vi "UHR-Fleezers Control (host) - 11.0.vi"() -> ()   [LabVIEW 2011] (continued)
                                }
                                frame #1 {
                                n486 = local read "Yank to which?"() -> (w782:bool)
                                n487 = case shown="False" w782 {
                                tunnel: w783 -> [_ w811]
                                tunnel: w781 -> [w784 _]
                                frame False {
                                n488 = flat-sequence {
                                tunnel: w784 -> [w785]
                                frame #0 {
                                n489 = property on="Trap Pos FB SP" class="DigNum (strict)"("Val(Sgnl)"=w785) -> ()  [unwired: 2 in, 2 out]
                                }
                                frame #1 {
                                n490 = Wait (ms)(milliseconds to wait=u32 700) -> ()  [unwired: 1 out]
                                }
                                frame #2 {
                                n491 = local read "Action (%)"() -> (w790:dbl)
                                n492 = Absolute Value(x=w790) -> (abs(x)=w789:dbl)
                                n493 = Greater?(x=w789, y=70.0) -> (0:w787:bool)
                                n494 = property on="Remove Action Offset" class="Bool (strict)"("Val(Sgnl)"=w787) -> ()  [unwired: 2 in, 2 out]
                                }
                                frame #3 {
                                n495 = for {
                                N: 4 -> [_]
                                n496 = flat-sequence {
                                frame #0 {
                                n497 = Wait (ms)(milliseconds to wait=u32 500) -> ()  [unwired: 1 out]
                                }
                                frame #1 {
                                n498 = local read "Action (%)"() -> (w796:dbl)
                                n499 = Absolute Value(x=w796) -> (abs(x)=w795:dbl)
                                n500 = Greater?(x=w795, y=70.0) -> (0:w793:bool)
                                n501 = property on="Remove Action Offset" class="Bool (strict)"("Val(Sgnl)"=w793) -> ()  [unwired: 2 in, 2 out]
                                }
                                }
                                }
                                }
                                frame #4 {
                                n502 = Wait (ms)(milliseconds to wait=u32 500) -> ()  [unwired: 1 out]
                                }
                                frame #5 {
                                n503 = local read "Shift confocal"() -> (w801:bool)
                                n504 = local read "Mean"() -> (w804:dbl)
                                n505 = Greater?(x=w804, y=11.0) -> (0:w800:bool)
                                n506 = Not(x=w800) -> (.not. x?=w799:bool)
                                n507 = And(x=w800, y=w801) -> (x .and. y?=w802:bool)
                                n508 = And(x=w799, y=w801) -> (x .and. y?=w798:bool)
                                n509 = case shown="True" w802 {
                                frame False {
                                }
                                frame True {
                                n510 = local read "Confocal X 2 (V)"() -> (w807:dbl)
                                n511 = local read "Confocal Y 2 (V)"() -> (w808:dbl)
                                n512 = property on="AO2" class="Slide (strict)"("Val(Sgnl)"=w807) -> ()  [unwired: 2 in, 2 out]
                                n513 = property on="AO1" class="Slide (strict)"("Val(Sgnl)"=w808) -> ()  [unwired: 2 in, 2 out]
                                }
                                }
                                n514 = case shown="True" w798 {
                                frame False {
                                }
                                frame True {
                                n515 = local read "Confocal Y 1 (V)"() -> (w806:dbl)
                                n516 = local read "Confocal X 1 (V)"() -> (w805:dbl)
                                n517 = property on="AO1" class="Slide (strict)"("Val(Sgnl)"=w806) -> ()  [unwired: 2 in, 2 out]
                                n518 = property on="AO2" class="Slide (strict)"("Val(Sgnl)"=w805) -> ()  [unwired: 2 in, 2 out]
                                }
                                }
                                }
                                frame #6 {
                                n519 = Wait (ms)(milliseconds to wait=u32 1500) -> ()  [unwired: 1 out]
                                }
                                frame #7 {
                                n520 = property on="Rem fb disp offset" class="Bool (strict)"("Val(Sgnl)"=TRUE ("Value (Signaling)")) -> ()  [unwired: 2 in, 2 out]
                                }
                                }
                                }
                                frame True {
                                n521 = flat-sequence {
                                tunnel: w811 -> [w812]
                                frame #0 {
                                n522 = property on="Trap Delta (MHz)" class="DigNum (strict)"("Val(Sgnl)"=w812) -> ()  [unwired: 2 in, 2 out]
                                }
                                frame #1 {
                                n523 = Wait (ms)(milliseconds to wait=u32 500) -> ()  [unwired: 1 out]
                                }
                                frame #2 {
                                n524 = local read "Shift confocal"() -> (w818:bool)
                                n525 = local read "Mean"() -> (w819:dbl)
                                n526 = Greater?(x=w819, y=11.0) -> (0:w817:bool)
                                n527 = And(x=w817, y=w818) -> (x .and. y?=w815:bool)
                                n528 = Not(x=w817) -> (.not. x?=w816:bool)
                                n529 = And(x=w816, y=w818) -> (x .and. y?=w814:bool)
                                n530 = case shown="True" w815 {
                                frame False {
                                }
                                frame True {
                                n531 = local read "Confocal Y 2 (V)"() -> (w824:dbl)
                                n532 = local read "Confocal X 2 (V)"() -> (w823:dbl)
                                n533 = property on="AO1" class="Slide (strict)"("Val(Sgnl)"=w824) -> ()  [unwired: 2 in, 2 out]
                                n534 = property on="AO2" class="Slide (strict)"("Val(Sgnl)"=w823) -> ()  [unwired: 2 in, 2 out]
                                }
                                }
                                n535 = case shown="True" w814 {
                                frame False {
                                }
                                frame True {
                                n536 = local read "Confocal Y 1 (V)"() -> (w822:dbl)
                                n537 = local read "Confocal X 1 (V)"() -> (w821:dbl)
                                n538 = property on="AO2" class="Slide (strict)"("Val(Sgnl)"=w821) -> ()  [unwired: 2 in, 2 out]
                                n539 = property on="AO1" class="Slide (strict)"("Val(Sgnl)"=w822) -> ()  [unwired: 2 in, 2 out]
                                }
                                }
                                }
                                }
                                }
                                }
                                }
                                }
                                }
                                }
                                n540 = local read "Time (s)"() -> (w759:dbl)
                                n541 = Subtract(x=w760, y=w759) -> (x-y=w771:dbl)
                                n542 = Number To Decimal String(number=w771, width (-)=i16 0) -> (decimal integer string=w769:string)
                                n543 = Concatenate Strings(w769, " s fluorescence event") -> (w766:string)
                                n544 = local read "Messages"() -> (w767:string)
                                n545 = local write "Duration (s)"(w771) -> ()
                                n546 = call "Update messages.vi"("Message to add"=w766, "Old message string"=w767) -> ("New message string"=w765:string)
                                n547 = local write "Messages"(w765) -> ()
                                n548 = call <vilib>:"Beep.vi"() -> ()  [unwired: 12 in]
                                n549 = local write "Reset Force"(FALSE ("Force Reset")) -> ()
                                n550 = local write "Fl. High"(TRUE ("Fl. High")) -> ()
                                n551 = local write "Waiting"(TRUE ("Waiting")) -> ()
                                }
                                }
                                n552 = node-c288() -> ()  [unwired: 1 in, 1 out]
                                }
                                n553 = node-c288(w738) -> ()  [unwired: 1 out]
                                }
                              }
                            }
                          }
                          n554 = local read "Trap Delta (MHz)"() -> (w650:dbl)
                          n555 = local read "Trap Pos FB SP"() -> (w648:fxp<+/-,16,1>)
                        }
                      }
                    }
                    frame True {
                      n556 = flat-sequence {
                        tunnel: w835 -> [w845]
                        tunnel: [w845] -> w839
                        tunnel: w838 -> [w844]
                        tunnel: [w844] -> w837
                        tunnel: [w843] -> w836
                        tunnel: w834 -> [w842]
                        tunnel: [w841] -> w833
                        tunnel: w830 -> [w840]
                        tunnel: [w840] -> w829
                        tunnel: w839 -> [w915]
                        tunnel: w837 -> [w914]
                        tunnel: w836 -> [w913]
                        tunnel: w833 -> [w912]
                        tunnel: w829 -> [w911]
                        tunnel: [w912] -> w832
                        frame #0 {
                          n557 = call <vilib>:"Beep.vi"() -> ()  [unwired: 3 in, 9 out]
                          n558 = local write "Waiting"(FALSE ("Waiting")) -> ()
                          n559 = Increment(x=w842) -> (x+1=w841:u8)
                          n560 = case shown="\"Yank\"" w844 {
                            tunnel: w841 -> [_ _ w851]
                            frame "Image" {
                              n561 = property on="Confocal Image" class="Bool (strict)"("Val(Sgnl)"=TRUE ("Value (Signaling)")) -> ()  [unwired: 2 in, 2 out]
                            }
                            frame "Alarm", Default {
                            }
                            frame "Yank" {
                              n562 = flat-sequence {
                                tunnel: w851 -> [w854]
                                tunnel: [w853] -> w850
                                tunnel: ["N Array El"] -> w849
                                tunnel: w850 -> [w868]
                                tunnel: w849 -> [w864]
                                frame #0 {
                                n563 = Multiply(x="Yank Delay (s)", y=1000.0) -> (x*y=w857:dbl)
                                n564 = Quotient & Remainder(x=w854, y="N Array El") -> (x-y*floor(x/y)=w853:u8)  [unwired: 1 out]
                                n565 = Wait (ms)(milliseconds to wait=w857) -> ()  [unwired: 1 out]
                                }
                                frame #1 {
                                n566 = Random Number (0-1)() -> (number: 0 to 1=w865:dbl)
                                n567 = Multiply(x=w864, y=w865) -> (x*y=w863:dbl)
                                n568 = Round Toward -Infinity(1:w863) -> (0:w862:dbl)
                                n569 = Select(t=w862, s="Random Choice", f=w868) -> (s? t:f=w866:dbl)
                                n570 = Select(t="Yank to Trap Delta (MHz)", s="Yank to which?", f="Yank to SP") -> (s? t:f=w859:dbl[])
                                n571 = Index Array(array=w859, index=w866) -> (element=w869:dbl)
                                n572 = case shown="False" "Yank to which?" {
                                tunnel: w869 -> [w870 w896]
                                frame False {
                                n573 = flat-sequence {
                                tunnel: w870 -> [w871]
                                frame #0 {
                                n574 = property on="Trap Pos FB SP" class="DigNum (strict)"("Val(Sgnl)"=w871) -> ()  [unwired: 2 in, 2 out]
                                }
                                frame #1 {
                                n575 = Wait (ms)(milliseconds to wait=u32 700) -> ()  [unwired: 1 out]
                                }
                                frame #2 {
                                n576 = local read "Action (%)"() -> (w876:dbl)
                                n577 = Absolute Value(x=w876) -> (abs(x)=w875:dbl)
                                n578 = Greater?(x=w875, y=70.0) -> (0:w873:bool)
                                n579 = property on="Remove Action Offset" class="Bool (strict)"("Val(Sgnl)"=w873) -> ()  [unwired: 2 in, 2 out]
                                }
                                frame #3 {
                                n580 = for {
                                N: 4 -> [_]
                                n581 = flat-sequence {
                                frame #0 {
                                n582 = Wait (ms)(milliseconds to wait=u32 500) -> ()  [unwired: 1 out]
                                }
                                frame #1 {
                                n583 = local read "Action (%)"() -> (w882:dbl)
                                n584 = Absolute Value(x=w882) -> (abs(x)=w881:dbl)
                                n585 = Greater?(x=w881, y=70.0) -> (0:w879:bool)
                                n586 = property on="Remove Action Offset" class="Bool (strict)"("Val(Sgnl)"=w879) -> ()  [unwired: 2 in, 2 out]
                                }
                                }
                                }
                                }
                                frame #4 {
                                n587 = local read "Shift confocal"() -> (w886:bool)
                                n588 = local read "Mean"() -> (w889:dbl)
                                n589 = Greater?(x=w889, y=11.0) -> (0:w885:bool)
                                n590 = Not(x=w885) -> (.not. x?=w884:bool)
                                n591 = And(x=w884, y=w886) -> (x .and. y?=w883:bool)
                                n592 = And(x=w885, y=w886) -> (x .and. y?=w887:bool)
                                n593 = case shown="True" w887 {
                                frame False {
                                }
                                frame True {
                                n594 = local read "Confocal X 2 (V)"() -> (w892:dbl)
                                n595 = local read "Confocal Y 2 (V)"() -> (w893:dbl)
                                n596 = property on="AO2" class="Slide (strict)"("Val(Sgnl)"=w892) -> ()  [unwired: 2 in, 2 out]
                                n597 = property on="AO1" class="Slide (strict)"("Val(Sgnl)"=w893) -> ()  [unwired: 2 in, 2 out]
                                }
                                }
                                n598 = case shown="True" w883 {
                                frame False {
                                }
                                frame True {
                                n599 = local read "Confocal X 1 (V)"() -> (w890:dbl)
                                n600 = local read "Confocal Y 1 (V)"() -> (w891:dbl)
                                n601 = property on="AO1" class="Slide (strict)"("Val(Sgnl)"=w891) -> ()  [unwired: 2 in, 2 out]
                                n602 = property on="AO2" class="Slide (strict)"("Val(Sgnl)"=w890) -> ()  [unwired: 2 in, 2 out]
                                }
                                }
                                }
                                frame #5 {
                                n603 = Wait (ms)(milliseconds to wait=u32 1500) -> ()  [unwired: 1 out]
                                }
                                frame #6 {
                                n604 = property on="Rem fb disp offset" class="Bool (strict)"("Val(Sgnl)"=TRUE ("Value (Signaling)")) -> ()  [unwired: 2 in, 2 out]
                                }
                                }
                                }
                                frame True {
                                n605 = flat-sequence {
                                tunnel: w896 -> [w897]
                                frame #0 {
                                n606 = property on="Trap Delta (MHz)" class="DigNum (strict)"("Val(Sgnl)"=w897) -> ()  [unwired: 2 in, 2 out]
                                }
                                frame #1 {
                                n607 = Wait (ms)(milliseconds to wait=u32 500) -> ()  [unwired: 1 out]
                                }
                                frame #2 {
                                n608 = local read "Shift confocal"() -> (w901:bool)
                                n609 = local read "Mean"() -> (w899:dbl)
                                n610 = Greater?(x=w899, y=11.0) -> (0:w902:bool)
                                n611 = Not(x=w902) -> (.not. x?=w903:bool)
                                n612 = And(x=w903, y=w901) -> (x .and. y?=w905:bool)
                                n613 = And(x=w902, y=w901) -> (x .and. y?=w904:bool)
                                n614 = case shown="True" w904 {
                                frame False {
                                }
                                frame True {
                                n615 = local read "Confocal Y 2 (V)"() -> (w909:dbl)
                                n616 = local read "Confocal X 2 (V)"() -> (w908:dbl)
                                n617 = property on="AO1" class="Slide (strict)"("Val(Sgnl)"=w909) -> ()  [unwired: 2 in, 2 out]
                                n618 = property on="AO2" class="Slide (strict)"("Val(Sgnl)"=w908) -> ()  [unwired: 2 in, 2 out]
                                }
                                }
                                n619 = case shown="True" w905 {
                                frame False {
                                }
                                frame True {
                                n620 = local read "Confocal X 1 (V)"() -> (w906:dbl)
                                n621 = local read "Confocal Y 1 (V)"() -> (w907:dbl)
                                n622 = property on="AO2" class="Slide (strict)"("Val(Sgnl)"=w906) -> ()  [unwired: 2 in, 2 out]
                                n623 = property on="AO1" class="Slide (strict)"("Val(Sgnl)"=w907) -> ()  [unwired: 2 in, 2 out]
                                }
                                }
                                }
                                }
                                }
                                }
                                }
                              }
                            }
                          }
                          n624 = local read "Time (s)"() -> (w843:dbl)
                          "Fl. High" <- TRUE ("Yanking")
                        }
                        frame #1 {
                          n625 = local read "Auto F Reset"() -> (w910:bool)
                          n626 = case shown="True" w910 {
                            tunnel: w915 -> [_ w919]
                            tunnel: w914 -> [_ w918]
                            tunnel: w913 -> [_ w917]
                            tunnel: w911 -> [_ w916]
                            frame False {
                            }
                            frame True {
                              n627 = node-c288() -> (w921:T21)  [unwired: 4 out]
                              n628 = timed-loop {
                                timing: w921 -> [_]
                                timing-out: [_] -> w920
                                tunnel: w919 -> [w939]
                                tunnel: w918 -> [w938]
                                tunnel: w917 -> [w937]
                                tunnel: w916 -> [w936]
                                stop <- w922 stop-if-true
                                n629 = node-c288() -> ()  [unwired: 2 out]
                                n630 = local read "Fl. Delta Thresh. (kHz)"() -> (w930:dbl)
                                n631 = local read "Fl. Triggered..."() -> (w935:bool)
                                n632 = local read "Delta Fl. 1"() -> (w926:dbl)
                                n633 = local read "Delta Fl. 2"() -> (w924:dbl)
                                n634 = local read "Stop All"() -> (w933:bool)
                                n635 = local read "APD to Watch"() -> (w925:bool)
                                n636 = Select(t=w926, s=w925, f=w924) -> (s? t:f=w923:dbl)
                                n637 = Not(x=w935) -> (.not. x?=w934:bool)
                                n638 = Multiply(x=w930, y=1000.0) -> (x*y=w929:dbl)
                                n639 = Negate(x=w929) -> (-x=w928:dbl)
                                n640 = Less?(x=w923, y=w928) -> (x < y?=w932:bool)
                                n641 = Compound Arithmetic op=OR(w932, w933, w934, "Reset Force") -> (w922:bool)
                                n642 = case shown="True" w922 {
                                tunnel: w939 -> [_ w954]
                                tunnel: w938 -> [_ w953]
                                tunnel: w937 -> [_ w943]
                                tunnel: w936 -> [_ w945]
                                frame False {
                                }
                                frame True {
                                n643 = local read "Time (s)"() -> (w944:dbl)
                                n644 = case shown="\"Yank\"" w953 {
                                tunnel: w954 -> [_ w957]
                                tunnel: w945 -> [_ w955]
                                frame "Image", Default {
                                }
                                frame "Yank" {
                                n645 = flat-sequence {
                                tunnel: [w963] -> w958
                                tunnel: w957 -> [w963]
                                tunnel: [w959] -> w956
                                tunnel: w955 -> [w959]
                                tunnel: w958 -> [w966]
                                tunnel: w956 -> [w964]
                                frame #0 {
                                n646 = local read "Yank Delay (s)"() -> (w962:dbl)
                                n647 = Multiply(x=w962, y=1000.0) -> (x*y=w960:dbl)
                                n648 = Wait (ms)(milliseconds to wait=w960) -> ()  [unwired: 1 out]
                                }
                                frame #1 {
                                n649 = local read "Yank to which?"() -> (w965:bool)
                                n650 = case shown="False" w965 {
                                tunnel: w966 -> [_ w993]
                                tunnel: w964 -> [w967 _]
                                frame False {
                                n651 = flat-sequence {
                                tunnel: w967 -> [w968]
                                frame #0 {
                                n652 = property on="Trap Pos FB SP" class="DigNum (strict)"("Val(Sgnl)"=w968) -> ()  [unwired: 2 in, 2 out]
                                }
                                frame #1 {
                                n653 = Wait (ms)(milliseconds to wait=u32 700) -> ()  [unwired: 1 out]
                                }
                                frame #2 {
                                n654 = local read "Action (%)"() -> (w973:dbl)
                                n655 = Absolute Value(x=w973) -> (abs(x)=w972:dbl)
                                n656 = Greater?(x=w972, y=70.0) -> (0:w970:bool)
                                n657 = property on="Remove Action Offset" class="Bool (strict)"("Val(Sgnl)"=w970) -> ()  [unwired: 2 in, 2 out]
                                }
                                frame #3 {
                                n658 = for {
                                N: 4 -> [_]
                                n659 = flat-sequence {
                                frame #0 {
                                n660 = Wait (ms)(milliseconds to wait=u32 500) -> ()  [unwired: 1 out]
                                }
                                frame #1 {
                                n661 = local read "Action (%)"() -> (w979:dbl)
                                n662 = Absolute Value(x=w979) -> (abs(x)=w978:dbl)
                                n663 = Greater?(x=w978, y=70.0) -> (0:w976:bool)
                                n664 = property on="Remove Action Offset" class="Bool (strict)"("Val(Sgnl)"=w976) -> ()  [unwired: 2 in, 2 out]
                                }
                                }
                                }
                                }
                                frame #4 {
                                n665 = local read "Shift confocal"() -> (w984:bool)
                                n666 = local read "Mean"() -> (w986:dbl)
                                n667 = Greater?(x=w986, y=11.0) -> (0:w983:bool)
                                n668 = Not(x=w983) -> (.not. x?=w982:bool)
                                n669 = And(x=w983, y=w984) -> (x .and. y?=w981:bool)
                                n670 = And(x=w982, y=w984) -> (x .and. y?=w980:bool)
                                n671 = case shown="True" w981 {
                                frame False {
                                }
                                frame True {
                                n672 = local read "Confocal Y 2 (V)"() -> (w990:dbl)
                                n673 = local read "Confocal X 2 (V)"() -> (w989:dbl)
                                n674 = property on="AO2" class="Slide (strict)"("Val(Sgnl)"=w989) -> ()  [unwired: 2 in, 2 out]
                                n675 = property on="AO1" class="Slide (strict)"("Val(Sgnl)"=w990) -> ()  [unwired: 2 in, 2 out]
                                }
                                }
                                n676 = case shown="True" w980 {
                                frame False {
                                }
                                frame True {
                                n677 = local read "Confocal X 1 (V)"() -> (w987:dbl)
                                n678 = local read "Confocal Y 1 (V)"() -> (w988:dbl)
                                n679 = property on="AO1" class="Slide (strict)"("Val(Sgnl)"=w988) -> ()  [unwired: 2 in, 2 out]
                                n680 = property on="AO2" class="Slide (strict)"("Val(Sgnl)"=w987) -> ()  [unwired: 2 in, 2 out]
                                }
                                }
                                }
                                frame #5 {
                                n681 = Wait (ms)(milliseconds to wait=u32 1500) -> ()  [unwired: 1 out]
                                }
                                frame #6 {
                                n682 = property on="Rem fb disp offset" class="Bool (strict)"("Val(Sgnl)"=TRUE ("Value (Signaling)")) -> ()  [unwired: 2 in, 2 out]
                                }
                                }
                                }
                                frame True {
                                n683 = flat-sequence {
                                tunnel: w993 -> [w994]
                                frame #0 {
                                n684 = property on="Trap Delta (MHz)" class="DigNum (strict)"("Val(Sgnl)"=w994) -> ()  [unwired: 2 in, 2 out]
                                }
                                frame #1 {
                                n685 = Wait (ms)(milliseconds to wait=u32 500) -> ()  [unwired: 1 out]
                                }
                                frame #2 {
                                n686 = local read "Shift confocal"() -> (w1000:bool)
                                n687 = local read "Mean"() -> (w1002:dbl)
                                n688 = Greater?(x=w1002, y=11.0) -> (0:w999:bool)
                                n689 = Not(x=w999) -> (.not. x?=w998:bool)
                                n690 = And(x=w999, y=w1000) -> (x .and. y?=w997:bool)
                                n691 = And(x=w998, y=w1000) -> (x .and. y?=w996:bool)
                                n692 = case shown="True" w997 {
                                frame False {
                                }
                                frame True {
                                n693 = local read "Confocal Y 2 (V)"() -> (w1006:dbl)
                                n694 = local read "Confocal X 2 (V)"() -> (w1005:dbl)
                                n695 = property on="AO2" class="Slide (strict)"("Val(Sgnl)"=w1005) -> ()  [unwired: 2 in, 2 out]
                                n696 = property on="AO1" class="Slide (strict)"("Val(Sgnl)"=w1006) -> ()  [unwired: 2 in, 2 out]
                                }
                                }
                                n697 = case shown="True" w996 {
                                frame False {
                                }
                                frame True {
                                n698 = local read "Confocal Y 1 (V)"() -> (w1004:dbl)
                                n699 = local read "Confocal X 1 (V)"() -> (w1003:dbl)
                                n700 = property on="AO2" class="Slide (strict)"("Val(Sgnl)"=w1003) -> ()  [unwired: 2 in, 2 out]
                                n701 = property on="AO1" class="Slide (strict)"("Val(Sgnl)"=w1004) -> ()  [unwired: 2 in, 2 out]
                                }
                                }
                                }
                                }
                                }
                                }
                                }
                                }
                                }
                                }
                                n702 = local read "Messages"() -> (w952:string)
                                n703 = Subtract(x=w944, y=w943) -> (x-y=w950:dbl)
                                "Duration (s)" <- w950
                                n704 = Number To Decimal String(number=w950, width (-)=i16 0) -> (decimal integer string=w948:string)
                                n705 = Concatenate Strings(w948, " s fluorescence event." ("string")) -> (w946:string)
                                n706 = call "Update messages.vi"("Message to add"=w946, "Old message string"=w952) -> ("New message string"=w951:string)
                                n707 = local write "Reset Force"(FALSE ("Reset Force")) -> ()
                                n708 = local write "Waiting"(TRUE ("Waiting")) -> ()
                                n709 = local write "Messages"(w951) -> ()
                                n710 = local write "Fl. High"(FALSE ("Fl. High")) -> ()
                                n711 = call <vilib>:"Beep.vi"() -> ()  [unwired: 3 in, 9 out]
                                }
                                }
                                n712 = node-c288() -> ()  [unwired: 2 out]
                              }
                              n713 = node-c288(w920) -> ()  [unwired: 1 out]
                            }
                          }
                        }
                      }
                      n714 = local read "Trap Delta (MHz)"() -> (w835:dbl)
                      n715 = local read "Trap Pos FB SP"() -> (w830:fxp<+/-,16,1>)
                    }
                  }
                }
                frame #1 {
                  n716 = local read "Stop All"() -> (w1016:bool)
                  n717 = local read "Fl. Triggered..."() -> (w1014:bool)
                  n718 = Not(x=w1014) -> (.not. x?=w1015:bool)
                  n719 = Or(x=w1015, y=w1016) -> (x .or. y?=w1013:bool)
                }
              }
              n720 = case shown="True" w607 {
                frame False {
                }
                frame True {
                  n721 = local read "Confocal Y 1 (V)"() -> (w617:dbl)
                  n722 = local read "Confocal X 1 (V)"() -> (w616:dbl)
                  n723 = property on="AO2" class="Slide (strict)"("Val(Sgnl)"=w616) -> ()  [unwired: 2 in, 2 out]
                  n724 = property on="AO1" class="Slide (strict)"("Val(Sgnl)"=w617) -> ()  [unwired: 2 in, 2 out]
                }
              }
              n725 = case shown="True" w607 {
                frame False {
                }
                frame True {
                  w615 = FALSE ("Fl. High")
                  n726 = local write "Waiting"(w615) -> ()
                  n727 = local write "Fl. High"(w615) -> ()
                }
              }
              n728 = node-c288() -> ()  [unwired: 2 out]
            }
            n729 = node-c288(w605) -> ()  [unwired: 1 out]
          }
        }
      }
      event "Stop All": Value Change {
        n730 = event-data() -> ()  [unwired: 7 out]
        n731 = local read "Stop All"() -> (w1021:bool)
      }
    }
    n732 = node-c288() -> ()  [unwired: 2 out]
  }
  n733 = node-c288() -> (w79:T21)  [unwired: 4 in]
  n734 = node-c288(2 ("Processor")) -> (w92:T21)  [unwired: 3 out]
  n735 = timed-loop "Run Scripts, including: stage motion" {
    tunnel: w84 -> [w1028]
    tunnel: w83 -> [w1029]
    tunnel: [w1029] -> w82
    tunnel: [w1028] -> w81
    timing: w79 -> [_]
    timing-out: [_] -> w78
    tunnel: w64 -> [w1027]
    tunnel: w65 -> [w1026]
    tunnel: w5 -> [w1023]
    tunnel: w4 -> [w1022]
    tunnel: w3 -> [w1024]
    tunnel: w2 -> [w1025]
    stop <- w1030 stop-if-true
    n736 = node-c288() -> ()  [unwired: 1 in, 1 out]
    n737 = event shown="[12] \"Force FB Data\nScript\": Value Change" {
      selector: _ -> [_ _ _ _ _ _ _ _ _ _ _ _ _ _ _ _ _ _ _]
      dyn-events: _ -> [_ _ _ _ _ _ _ _ _ _ _ _ _ _ _ _ _ _ _]
      timeout: _ -> [_ _ _ _ _ _ _ _ _ _ _ _ _ _ _ _ _ _ _]
      tunnel: ["Set Position" "Move to Position" _ _ "Read Harvard" _ _ _ _ _ _ "Got ADig bead" "Force FB Data\nScript" _ "Got DNA bead" "Take Stepping Data" _ "Take Detection Laser\nImage" _] -> _
      tunnel: [_ _ _ _ _ _ _ _ _ _ _ _ _ _ _ _ _ _ w1647] -> w1030
      tunnel: w1028 -> [w1048 w1056 w1069 w1099 _ w1144 w1184 w1265 w1294 w1426 w1452 _ w1488 _ _ _ _ _ _]
      tunnel: w1029 -> [w1049 w1057 w1070 w1100 _ w1145 w1185 w1266 w1295 w1427 w1453 _ w1489 _ _ _ _ _ _]
      tunnel: w1027 -> [_ _ _ _ w1129 _ _ _ _ _ _ _ _ _ _ _ _ _ _]
      tunnel: w1026 -> [_ _ _ _ w1128 _ _ _ _ _ _ _ _ _ _ _ _ _ _]
      tunnel: w1025 -> [_ _ _ _ _ _ _ _ _ _ _ _ _ _ _ _ _ _ _]
      tunnel: w1024 -> [_ _ _ _ _ _ _ _ _ _ _ _ _ _ _ _ _ _ _]
      tunnel: w1023 -> [_ _ _ _ _ _ _ _ _ _ _ _ _ _ _ _ _ _ _]
      tunnel: w1022 -> [_ _ _ _ _ _ _ _ _ _ _ _ _ _ _ _ _ _ _]
      event "Set Position", "Set Position 2", "Set Position 3", "Set Position 4", "Set Position 5", "Set Position 1": Value Change {
        n738 = event-data() -> ()  [unwired: 1 in, 5 out]
        n739 = Build Array("Set Position 1", "Set Position 2", "Set Position 3", "Set Position 4", "Set Position 5") -> (w1047:bool[])
        n740 = Boolean Array To Number(Boolean array=w1047) -> (number=w1046:u32)
        n741 = Logarithm Base 2(1:w1046) -> (0:w1038:dbl)
        n742 = call "Read Stage Position.vi"("error in"=w1048, "VISA resource name in"=w1049) -> ("Current Position"=w1053:cluster{dbl, dbl, dbl}, "error out"=w1052:errorcluster)  [unwired: 2 out]
        n743 = Decrement(x="Position") -> (x-1=w1036:dbl)
        n744 = Greater Or Equal?(x=w1038, y=0.0) -> (x >= y?=w1039:bool)
        n745 = Cluster To Array(cluster=w1053) -> (array=w1050:dbl[])
        n746 = local write "Stage Control Serial Error"(w1052) -> ()
        n747 = Select(t=w1038, s=w1039, f=w1036) -> (s? t:f=w1035:dbl)
        n748 = Increment(x=w1035) -> (x+1=w1034:dbl)
        n749 = Build Array (concatenate)(w1034, w1050) -> (w1033:dbl[])
        n750 = Replace Array Subset(array="Saved Stage Positions", new element=w1033, index (row)=w1035) -> (w1051:dbl[][])  [unwired: 1 in]
        n751 = local write "Saved Stage Positions"(w1051) -> ()
      }
      event "Move to Position": Value Change {
        n752 = event-data() -> ()  [unwired: 1 in, 5 out]
        n753 = flat-sequence {
          tunnel: w1057 -> [w1061]
          tunnel: w1056 -> [w1060]
          frame #0 {
            n754 = local read "Saved Stage Positions"() -> (w1063:dbl[][])
            n755 = local read "Position"() -> (w1062:dbl)
            n756 = local write "Stage Moving"(TRUE ("Stage Moving")) -> ()
            n757 = call "move to saved stage position.vi"("error in"=w1060, "Stage VISA resource name in"=w1061, "Position"=w1062, "Saved Stage Positions"=w1063) -> ("error out"=w1059:errorcluster)  [unwired: 1 out]
            n758 = local write "Stage Control Serial Error"(w1059) -> ()
          }
          frame #1 {
            n759 = call <vilib>:"Beep.vi"() -> ()  [unwired: 3 in, 9 out]
            n760 = local write "Stage Moving"(FALSE ("Stage Moving")) -> ()
          }
        }
      }
      event "Move Cap. 1 (DNA Bottom)": Value Change {
        n761 = event-data() -> ()  [unwired: 1 in, 5 out]
        n762 = local write "Move Cap. 1 (DNA Bottom)"(FALSE ("Move Cap. 1 (DNA Right)")) -> ()
        n763 = flat-sequence {
          tunnel: w1069 -> [w1072]
          tunnel: w1070 -> [w1073]
          tunnel: [w1073] -> w1067
          tunnel: [w1072] -> w1066
          tunnel: w1067 -> [w1075]
          tunnel: w1066 -> [w1074]
          frame #0 {
            n764 = property on="Sample Channel\nFlow" class="Bool (strict)"("Val(Sgnl)"="Cap 1 Samp Flow ON") -> ()  [unwired: 2 in, 2 out]
          }
          frame #1 {
            n765 = local read "Saved Stage Positions"() -> (w1085:dbl[][])
            n766 = local write "Stage Moving"(TRUE ("Stage Moving")) -> ()
            n767 = Array Subset(array=w1085, index (row)=0 ("index"), length (row)=1 ("length"), index (col)=1 ("index"), length (col)=3 ("length")) -> (w1082:dbl[][])
            n768 = Reshape Array(w1082, 3 ("dimension size")) -> (w1080:dbl[])
            n769 = Array To Cluster(array=w1080) -> (cluster=w1079:cluster{"[0]":dbl, "[1]":dbl, "[2]":dbl})
            n770 = call "Set Stage Position.vi"("Position"=w1079, "error in"=w1074, "VISA resource name in"=w1075) -> ("error out"=w1078:errorcluster)  [unwired: 2 out]
            n771 = local write "Stage Control Serial Error"(w1078) -> ()
          }
          frame #2 {
            n772 = local write "Stage Moving"(FALSE ("Stage Moving")) -> ()
            n773 = case shown="True" "Cap 1 Flow ON" {
              frame False {
              }
              frame True {
                n774 = property on="Inject Pump 1" class="Bool (strict)"("Val(Sgnl)"=TRUE ("Value (Signaling)")) -> ()  [unwired: 2 in, 2 out]
              }
            }
            n775 = call <vilib>:"Beep.vi"() -> ()  [unwired: 3 in, 9 out]
          }
          frame #3 {
            n776 = property on="Sample Channel\nFlow" class="Bool (strict)"("Val(Sgnl)"=FALSE ("Value (Signaling)")) -> ()  [unwired: 2 in, 2 out]
            n777 = local read "Cap. 2 BD T1?\n(ADig T1, DNA T2)"() -> (w1092:bool)
            n778 = case shown="True" w1092 {
              tunnel: "Cap 1 T ON" -> [w1094 w1095]
              frame False {
                n779 = property on="Trap 1 (ON/OFF)" class="Bool (strict)"("Val(Sgnl)"=w1094) -> ()  [unwired: 2 in, 2 out]
              }
              frame True {
                n780 = property on="Trap 2 (ON/OFF)" class="Bool (strict)"("Val(Sgnl)"=w1095) -> ()  [unwired: 2 in, 2 out]
              }
            }
            n781 = property on="Got DNA bead" class="Bool"("Key Focus"=TRUE) -> ()  [unwired: 2 in, 2 out]
          }
        }
      }
      event "Move Cap. 2 (ADig Top)": Value Change {
        n782 = event-data() -> ()  [unwired: 1 in, 5 out]
        n783 = local write "Move Cap. 2 (ADig Top)"(FALSE ("Move Cap. 2 (ADig Left)")) -> ()
        n784 = flat-sequence {
          tunnel: w1099 -> [w1102]
          tunnel: w1100 -> [w1103]
          tunnel: [w1103] -> w1097
          tunnel: [w1102] -> w1096
          tunnel: w1097 -> [w1106]
          tunnel: w1096 -> [w1105]
          frame #0 {
            n785 = property on="Sample Channel\nFlow" class="Bool (strict)"("Val(Sgnl)"="Cap 2 Samp Flow ON") -> ()  [unwired: 2 in, 2 out]
          }
          frame #1 {
            w1104 = FALSE ("Value (Signaling)")
            n786 = local read "Saved Stage Positions"() -> (w1116:dbl[][])
            n787 = local write "Stage Moving"(TRUE ("Stage Moving")) -> ()
            n788 = Array Subset(array=w1116, index (row)=1 ("index"), length (row)=1 ("length"), index (col)=1 ("index"), length (col)=3 ("length")) -> (w1113:dbl[][])
            n789 = Reshape Array(w1113, 3 ("dimension size")) -> (w1111:dbl[])
            n790 = property on="Trap 1 (ON/OFF)" class="Bool (strict)"("Val(Sgnl)"=w1104) -> ()  [unwired: 2 in, 2 out]
            n791 = property on="Trap 1 (ON/OFF)" class="Bool (strict)"("Val(Sgnl)"=w1104) -> ()  [unwired: 2 in, 2 out]
            n792 = Array To Cluster(array=w1111) -> (cluster=w1110:cluster{"[0]":dbl, "[1]":dbl, "[2]":dbl})
            n793 = call "Set Stage Position.vi"("Position"=w1110, "error in"=w1105, "VISA resource name in"=w1106) -> ("error out"=w1109:errorcluster)  [unwired: 2 out]
            n794 = local write "Stage Control Serial Error"(w1109) -> ()
          }
          frame #2 {
            n795 = local write "Stage Moving"(FALSE ("Stage Moving")) -> ()
            n796 = call <vilib>:"Beep.vi"() -> ()  [unwired: 3 in, 9 out]
            n797 = case shown="True" "Cap 2 Flow ON" {
              frame False {
              }
              frame True {
                n798 = property on="Inject Pump 3" class="Bool (strict)"("Val(Sgnl)"=TRUE ("Value (Signaling)")) -> ()  [unwired: 2 in, 2 out]
              }
            }
          }
          frame #3 {
            n799 = property on="Sample Channel\nFlow" class="Bool (strict)"("Val(Sgnl)"=FALSE ("Value (Signaling)")) -> ()  [unwired: 2 in, 2 out]
            n800 = case shown="False" "Cap. 2 BD T1?\n(ADig T1, DNA T2)" {
              tunnel: "Cap 2 T ON" -> [w1125 w1126]
              frame False {
                n801 = property on="Trap 2 (ON/OFF)" class="Bool (strict)"("Val(Sgnl)"=w1125) -> ()  [unwired: 2 in, 2 out]
              }
              frame True {
                n802 = property on="Trap 1 (ON/OFF)" class="Bool (strict)"("Val(Sgnl)"=w1126) -> ()  [unwired: 2 in, 2 out]
              }
            }
            n803 = property on="Got ADig bead" class="Bool"("Key Focus"=TRUE) -> ()  [unwired: 2 in, 2 out]
          }
        }
      }
      event "Read Harvard": Value Change {
        n804 = event-data() -> ()  [unwired: 1 in, 5 out]
        n805 = Concatenate Strings("write buffer", "\r") -> (w1131:string)
        n806 = VISA Write(VISA resource name=w1129, write buffer=w1131, error in (no error)=w1128) -> (VISA resource name out=w1140:refnum<visa-resource-name>, error out=w1139:errorcluster)  [unwired: 1 out]
        n807 = stacked-sequence {
          tunnel: [w1143] -> w1138
          tunnel: w1140 -> [w1143]
          tunnel: w1139 -> [w1142]
          tunnel: [w1142] -> w1133
          frame #0 {
            n808 = Wait (ms)(milliseconds to wait=50) -> ()  [unwired: 1 out]
          }
        }
        n809 = property class="Instr"(reference=w1138, error in=w1133) -> (reference out=w1137:refnum<visa-resource-name>, error out=w1135:errorcluster, "Serial Settings:Number of Bytes at Serial Port"=w1136:u32)
        "Serial Settings:Number of Bytes at Serial Port" <- w1136
        n810 = VISA Read(VISA resource name=w1137, byte count=w1136, error in (no error)=w1135) -> (read buffer=w1134:string)  [unwired: 3 out]
        "read buffer" <- w1134
        n811 = Fract/Exp String To Number(string=w1134) -> ()  [unwired: 5 out]
      }
      event "+z", "-z": Value Change {
        n812 = event-data() -> ()  [unwired: 1 in, 5 out]
        n813 = flat-sequence {
          tunnel: w1144 -> [w1166]
          tunnel: w1145 -> [w1146]
          frame #0 {
            n814 = call "Read Stage Position.vi"("error in"=w1166, "VISA resource name in"=w1146) -> ("Current Position"=w1151:cluster{dbl, dbl, dbl}, "error out"=w1164:errorcluster, "VISA resource name out"=w1165:refnum<visa-resource-name>)  [unwired: 1 out]
            n815 = local read "Saved Stage Positions"() -> (w1175:dbl[][])
            n816 = Divide(x="z nudge increment (um)", y=1000.0) -> (x/y=w1163:dbl)
            n817 = Boolean To (0,1)(Boolean="+z") -> (0, 1=w1155:i16)
            n818 = Boolean To (0,1)(Boolean="-z") -> (0, 1=w1156:i16)
            n819 = Array Subset(array=w1175, index (row)=1 ("index"), length (row)=1 ("length"), index (col)=1 ("index"), length (col)=3 ("length")) -> (w1172:dbl[][])
            n820 = Multiply(x=w1155, y=w1163) -> (x*y=w1159:dbl)
            n821 = Multiply(x=w1156, y=w1163) -> (x*y=w1157:dbl)
            n822 = Unbundle(w1151) -> (w1149:dbl, w1148:dbl, w1152:dbl)
            n823 = Negate(x=w1157) -> (-x=w1158:dbl)
            n824 = Reshape Array(w1172, 3 ("dimension size")) -> (w1170:dbl[])
            n825 = Add(x=w1159, y=w1158) -> (x+y=w1160:dbl)
            n826 = Array To Cluster(array=w1170) -> ()  [unwired: 1 out]
            n827 = Add(x=w1160, y=w1152) -> (x+y=w1150:dbl)
            n828 = Bundle(cluster=w1151, w1149, w1148, w1150) -> (w1147:cluster{dbl, dbl, dbl})
            n829 = call "Set Stage Position.vi"("Position"=w1147, "error in"=w1164, "VISA resource name in"=w1165) -> ("error out"=w1169:errorcluster)  [unwired: 2 out]
            n830 = local write "Stage Moving"(TRUE ("Stage Moving")) -> ()
            n831 = local write "Stage Control Serial Error"(w1169) -> ()
          }
          frame #1 {
            n832 = local write "Stage Moving"(FALSE ("Stage Moving")) -> ()
            n833 = call <vilib>:"Beep.vi"() -> ()  [unwired: 3 in, 9 out]
          }
        }
      }
      event "Cal/Data Acq. Spot": Value Change {
        n834 = event-data() -> ()  [unwired: 1 in, 5 out]
        n835 = flat-sequence {
          tunnel: w1184 -> [w1188]
          tunnel: w1185 -> [w1189]
          tunnel: [w1189] -> w1181
          tunnel: [w1188] -> w1180
          tunnel: w1181 -> [w1194]
          tunnel: w1180 -> [w1193]
          tunnel: ["Cal @ (MHz)"] -> w1178
          tunnel: [w1198] -> w1182
          tunnel: w1178 -> [w1198]
          tunnel: w1182 -> [w1207]
          tunnel: ["W/ Offset 1"] -> w1179
          tunnel: w1182 -> [w1228]
          tunnel: w1179 -> [w1226]
          frame #0 {
            n836 = property on="Sample Channel\nFlow" class="Bool (strict)"("Val(Sgnl)"="Daq spot flow on") -> ()  [unwired: 2 in, 2 out]
            n837 = Wait (ms)(milliseconds to wait=u32 250) -> ()  [unwired: 1 out]
          }
          frame #1 {
            n838 = local read "Saved Stage Positions"() -> (w1191:dbl[][])
            n839 = property on="Trap Delta (MHz)" class="DigNum (strict)"("Val(Sgnl)"="Cal @ (MHz)") -> ()  [unwired: 2 in, 2 out]
            n840 = local write "Stage Moving"(TRUE ("Stage Moving")) -> ()
            n841 = call "move to saved stage position.vi"("error in"=w1193, "Stage VISA resource name in"=w1194, "Position"="Cal Stage Position", "Saved Stage Positions"=w1191) -> ("error out"=w1192:errorcluster)  [unwired: 1 out]
            n842 = local write "Stage Control Serial Error"(w1192) -> ()
          }
          frame #2 {
            n843 = local write "Stage Moving"(FALSE ("Stage Moving")) -> ()
            n844 = property on="Sample Channel\nFlow" class="Bool (strict)"("Val(Sgnl)"="Flow ON during cal?") -> ()  [unwired: 2 in, 2 out]
            n845 = call <vilib>:"Beep.vi"() -> ()  [unwired: 3 in, 9 out]
          }
          frame #3 {
            n846 = Wait (ms)(milliseconds to wait=u32 1000) -> ()  [unwired: 1 out]
          }
          frame #4 {
            n847 = property on="Save Calibration" class="Bool (strict)"("Val(Sgnl)"=TRUE ("Value (Signaling)")) -> ()  [unwired: 2 in, 2 out]
          }
          frame #5 {
            n848 = Wait (ms)(milliseconds to wait=u32 2000) -> ()  [unwired: 1 out]
          }
          frame #6 {
            # "Check to see if \nsaving done"
            n849 = while {
              stop <- w1203 stop-if-true
              n850 = local read "Saving..."() -> (w1204:bool)
              n851 = Wait (ms)(milliseconds to wait=u32 100) -> ()  [unwired: 1 out]
              n852 = Not(x=w1204) -> (.not. x?=w1203:bool)
            }
          }
          frame #7 {
            n853 = case shown="True" "W/ Offset 1" {
              tunnel: w1207 -> [_ w1208]
              frame False {
              }
              frame True {
                n854 = stacked-sequence {
                  tunnel: w1208 -> [_ _ _ _ _ _ _ w1225]
                  frame #0 {
                    n855 = property on="Trap Delta (MHz)" class="DigNum (strict)"("Val(Sgnl)"="Offset 1 Start (MHz)") -> ()  [unwired: 2 in, 2 out]
                    n856 = Replace Array Subset(array=u32[] [0] ("Index Values"), new element="Offset 1 Set", index=0) -> (w1209:u32[])
                    n857 = property on="Saved AOD Raster Scan Parameter Sets" class="Arr (strict)"("Index Values"=w1209) -> ()  [unwired: 2 in, 2 out]
                  }
                  frame #1 {
                    n858 = Wait (ms)(milliseconds to wait=u32 200) -> ()  [unwired: 1 out]
                  }
                  frame #2 {
                    n859 = property on="Load parameters" class="Bool (strict)"("Val(Sgnl)"=TRUE ("Value (Signaling)")) -> ()  [unwired: 2 in, 2 out]
                  }
                  frame #3 {
                    n860 = Wait (ms)(milliseconds to wait=u32 200) -> ()  [unwired: 1 out]
                  }
                  frame #4 {
                    n861 = property on="Trap Raster Scan" class="Bool (strict)"("Val(Sgnl)"=TRUE ("Value (Signaling)")) -> ()  [unwired: 2 in, 2 out]
                  }
                  frame #5 {
                    n862 = Wait (ms)(milliseconds to wait=u32 2000) -> ()  [unwired: 1 out]
                  }
                  frame #6 {
                    n863 = while {
                      stop <- w1222 stop-if-true
                      n864 = local read "Raster Scanning..."() -> (w1224:bool)
                      n865 = local read "Saving..."() -> (w1220:bool)
                      n866 = Wait (ms)(milliseconds to wait=u32 100) -> ()  [unwired: 1 out]
                      n867 = Not(x=w1220) -> (.not. x?=w1219:bool)
                      n868 = Not(x=w1224) -> (.not. x?=w1221:bool)
                      n869 = And(x=w1221, y=w1219) -> (x .and. y?=w1222:bool)
                    }
                  }
                  frame #7 {
                    n870 = property on="Trap Delta (MHz)" class="DigNum (strict)"("Val(Sgnl)"=w1225) -> ()  [unwired: 2 in, 2 out]
                  }
                }
              }
            }
          }
          frame #8 {
            n871 = local read "Save ave N"() -> (w1227:dbl)
            n872 = case shown="False" "W/ Offset 2" {
              tunnel: w1228 -> [_ w1235]
              tunnel: w1227 -> [_ w1234]
              tunnel: w1226 -> [w1230 _]
              frame False {
                n873 = case shown="False" w1230 {
                  frame False {
                    n874 = Multiply(x="Cal read wait (s)", y=u32 1000 ("milliseconds to wait")) -> (x*y=w1232:u32)
                    n875 = Wait (ms)(milliseconds to wait=w1232) -> ()  [unwired: 1 out]
                  }
                  frame True {
                  }
                }
              }
              frame True {
                n876 = stacked-sequence {
                  tunnel: w1235 -> [_ _ _ _ _ _ _ _ _ w1256 _ _]
                  tunnel: w1234 -> [_ _ _ _ _ _ _ _ _ w1254 _ _]
                  frame #0 {
                    n877 = property on="Save ave N" class="DigNum (strict)"("Val(Sgnl)"=1.0 ("Value (Signaling)")) -> ()  [unwired: 2 in, 2 out]
                  }
                  frame #1 {
                    n878 = Wait (ms)(milliseconds to wait=u32 500) -> ()  [unwired: 1 out]
                  }
                  frame #2 {
                    n879 = property on="Trap Delta (MHz)" class="DigNum (strict)"("Val(Sgnl)"="Offset 2 Start (MHz)") -> ()  [unwired: 2 in, 2 out]
                    n880 = Replace Array Subset(array=u32[] [0] ("Index Values"), new element="Offset 2 Set", index=0) -> (w1240:u32[])
                    n881 = property on="Saved AOD Raster Scan Parameter Sets" class="Arr (strict)"("Index Values"=w1240) -> ()  [unwired: 2 in, 2 out]
                  }
                  frame #3 {
                    n882 = Wait (ms)(milliseconds to wait=u32 500) -> ()  [unwired: 1 out]
                  }
                  frame #4 {
                    n883 = property on="Load parameters" class="Bool (strict)"("Val(Sgnl)"=TRUE ("Value (Signaling)")) -> ()  [unwired: 2 in, 2 out]
                  }
                  frame #5 {
                    n884 = Wait (ms)(milliseconds to wait=u32 500) -> ()  [unwired: 1 out]
                  }
                  frame #6 {
                    n885 = property on="Trap Raster Scan" class="Bool (strict)"("Val(Sgnl)"=TRUE ("Value (Signaling)")) -> ()  [unwired: 2 in, 2 out]
                  }
                  frame #7 {
                    n886 = Wait (ms)(milliseconds to wait=u32 2000) -> ()  [unwired: 1 out]
                  }
                  frame #8 {
                    n887 = while {
                      stop <- w1249 stop-if-true
                      n888 = local read "Raster Scanning..."() -> (w1252:bool)
                      n889 = local read "Saving..."() -> (w1250:bool)
                      n890 = Wait (ms)(milliseconds to wait=u32 100) -> ()  [unwired: 1 out]
                      n891 = Not(x=w1250) -> (.not. x?=w1248:bool)
                      n892 = Not(x=w1252) -> (.not. x?=w1251:bool)
                      n893 = And(x=w1251, y=w1248) -> (x .and. y?=w1249:bool)
                    }
                  }
                  frame #9 {
                    n894 = property on="Trap Delta (MHz)" class="DigNum (strict)"("Val(Sgnl)"=w1256) -> ()  [unwired: 2 in, 2 out]
                    n895 = property on="Saved AOD Raster Scan Parameter Sets" class="Arr (strict)"("Index Values"=u32[] [0]) -> ()  [unwired: 2 in, 2 out]
                    n896 = property on="Save ave N" class="DigNum (strict)"("Val(Sgnl)"=w1254) -> ()  [unwired: 2 in, 2 out]
                  }
                  frame #10 {
                    n897 = Wait (ms)(milliseconds to wait=u32 500) -> ()  [unwired: 1 out]
                  }
                  frame #11 {
                    n898 = property on="Load parameters" class="Bool (strict)"("Val(Sgnl)"=TRUE ("Value (Signaling)")) -> ()  [unwired: 2 in, 2 out]
                  }
                }
              }
            }
          }
          frame #9 {
            n899 = property on="Read Cal" class="Bool (strict)"("Val(Sgnl)"=TRUE ("Value (Signaling)")) -> ()  [unwired: 2 in, 2 out]
          }
          frame #10 {
            n900 = Wait (ms)(milliseconds to wait=u32 1000) -> ()  [unwired: 1 out]
          }
          frame #11 {
            n901 = property on="Fish for Tether" class="Bool (strict)"("Val(Sgnl)"=TRUE ("Value (Signaling)")) -> ()  [unwired: 2 in, 2 out]
          }
        }
        n902 = local write "Cal/Data Acq. Spot"(FALSE ("Cal/Data Acq. Spot")) -> ()
      }
      event "Dump Beads": Value Change {
        n903 = event-data() -> ()  [unwired: 1 in, 5 out]
        n904 = flat-sequence {
          tunnel: ["Dump spot flow on?"] -> w1262
          tunnel: [w1273] -> w1263
          tunnel: w1262 -> [w1273]
          tunnel: w1266 -> [w1278]
          tunnel: w1265 -> [w1277]
          tunnel: [w1275] -> w1264
          tunnel: w1263 -> [w1275]
          tunnel: w1264 -> [w1288]
          frame #0 {
            w1267 = FALSE ("Value (Signaling)")
            n905 = local read "Saving..."() -> (w1269:bool)
            n906 = local write "Dump Beads"(FALSE ("Dump Beads")) -> ()
            n907 = property on="Inject Pump 3" class="Bool (strict)"("Val(Sgnl)"=w1267) -> ()  [unwired: 2 in, 2 out]
            n908 = property on="Inject Pump 1" class="Bool (strict)"("Val(Sgnl)"=w1267) -> ()  [unwired: 2 in, 2 out]
            n909 = local write "Stop Saving"(w1269) -> ()
          }
          frame #1 {
            w1270 = FALSE ("Fl. Triggered...")
            n910 = case shown="True" "Dump spot flow on?" {
              frame False {
              }
              frame True {
                n911 = property on="Sample Channel\nFlow" class="Bool (strict)"("Val(Sgnl)"=TRUE ("Stage Moving")) -> ()  [unwired: 2 in, 2 out]
              }
            }
            n912 = local write "Fl. Triggered..."(w1270) -> ()
            n913 = local write "Tether"(w1270) -> ()
            n914 = property on="Green Laser ON/Interlacing" class="Bool (strict)"("Val(Sgnl)"=w1270) -> ()  [unwired: 2 in, 2 out]
            n915 = property on="Trap Pos. FB ON" class="Bool (strict)"("Val(Sgnl)"=w1270) -> ()  [unwired: 2 in, 2 out]
            n916 = property on="Trap Trig. Fl." class="Bool (strict)"("Val(Sgnl)"=w1270) -> ()  [unwired: 2 in, 2 out]
            n917 = property on="Fl. Triggered..." class="Bool (strict)"("Val(Sgnl)"=w1270) -> ()  [unwired: 2 in, 2 out]
            n918 = property on="Dip for Protein" class="Bool (strict)"("Val(Sgnl)"=w1270) -> ()  [unwired: 2 in, 2 out]
            n919 = property on="Pause dwell" class="Bool (strict)"("Val(Sgnl)"=w1270) -> ()  [unwired: 2 in, 2 out]
          }
          frame #2 {
            n920 = property on="Trap Pos. FB Offset Factor" class="DigNum (strict)"("Val(Sgnl)"=i64 0 ("Value (Signaling)")) -> ()  [unwired: 2 in, 2 out]
          }
          frame #3 {
            n921 = local read "Saved Stage Positions"() -> (w1279:dbl[][])
            n922 = local write "Stage Moving"(TRUE ("Stage Moving")) -> ()
            n923 = Array Subset(array=w1279, index (row)=3 ("index"), length (row)=1 ("length"), index (col)=1 ("index"), length (col)=3 ("length")) -> (w1284:dbl[][])
            n924 = Reshape Array(w1284, 3 ("dimension size")) -> (w1282:dbl[])
            n925 = Array To Cluster(array=w1282) -> (cluster=w1281:cluster{"[0]":dbl, "[1]":dbl, "[2]":dbl})
            n926 = call "Set Stage Position.vi"("Position"=w1281, "error in"=w1277, "VISA resource name in"=w1278) -> ()  [unwired: 3 out]
          }
          frame #4 {
